vi "Set SigGen Parameters.vi"(6 "Cal Route":string[](array[string])=["", "", ""], 7 "Cal?":bool, 8 "error in (no error)":errorcluster, 9 "Frequency (Hz)":dbl=100000000.0 format="%.3p", 10 "Amplitude":dbl format="%.2f", 11 "VISA Refnum in":refnum<visa-resource-name>) -> (0 "error out":errorcluster, 2 "Adjusted Power Level":dbl, 3 "VISA Refnum out":refnum<visa-resource-name>)   [LabVIEW 2015]
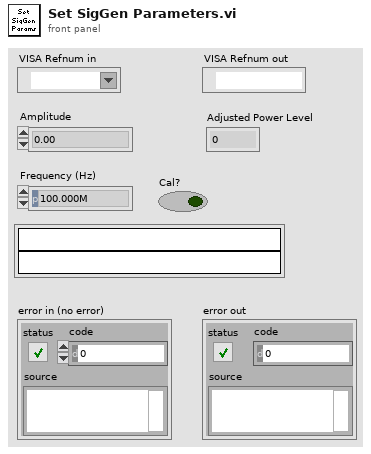
[diagram p1: front panel]
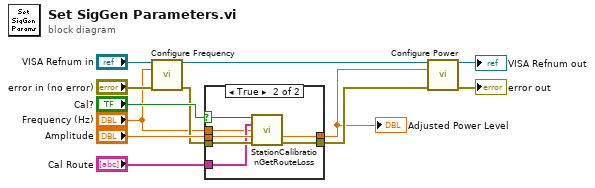
[diagram p0: block diagram]
diagram:
  n1 = call <instrlib>:"Configure Frequency.vi"("VISA resource name"="VISA Refnum in", "Frequency (100 kHz)"="Frequency (Hz)", "error in (no error)"="error in (no error)") -> ("VISA resource name out"=w10:refnum<visa-resource-name>, "error out"=w4:errorcluster)  [unwired: 11 in]
  n2 = case shown="True" "Cal?" {
    selector: "Cal?" -> [_ w15]
    tunnel: [w13 w21] -> w2
    tunnel: [w14 w16] -> w3
    tunnel: w4 -> [w14 w20]
    tunnel: "Amplitude" -> [w13 w19]
    tunnel: "Cal Route" -> [_ w18]
    tunnel: "Frequency (Hz)" -> [_ w17]
    frame False {
    }
    frame True {
      n3 = call "StationCalibrationGetRouteLoss.vi"("Calibration Enabled"=w15, "Route Names"=w18, "Frequency"=w17, "Power Level"=w19, "error in (no error)"=w20) -> ("Adjusted Power Level"=w21:dbl, "error out"=w16:errorcluster)  [unwired: 7 in, 2 out]
    }
  }
  "Adjusted Power Level" <- w2
  n4 = call <instrlib>:"Configure Power.vi"("VISA resource name"=w10, "Power (-130 dBm)"=w2, "error in (no error)"=w3) -> ("VISA resource name out"=→"VISA Refnum out":refnum<visa-resource-name>, "error out"=→"error out":errorcluster)  [unwired: 11 in]
